vi "add to buffer.vi"(10 "read data":string, 11 "buffer in":cluster{"data":u8[], "packets contained":i32}[](array[cluster])) -> (3 "buffer out":cluster{"data":u8[], "packets contained":i32}[](array[cluster]))   [LabVIEW 2020, in "SubVIs.lvlib" / "RTU Data Unit.lvclass"]
uses:
  <vilib>/Modbus/subvis/Transmission Data Unit (ADU)/RTU Data Unit/RTU Data Unit.lvclass
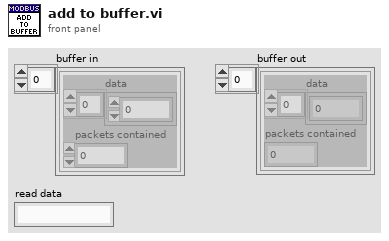
[diagram p1: front panel]
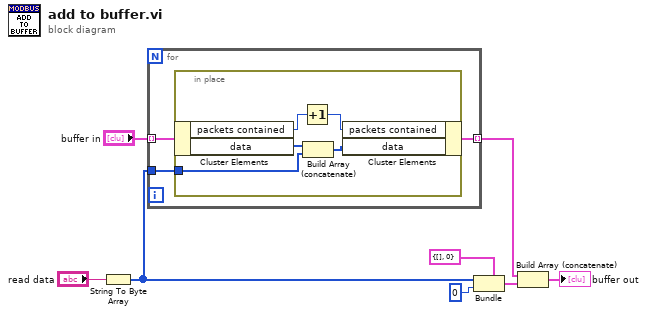
[diagram p0: block diagram]
diagram:
  n1 = String To Byte Array(string="read data") -> (unsigned byte array=w3:u8[])
  n2 = for {
    tunnel: "buffer in" -> [w11] mode=indexing
    tunnel: [w10] -> w4 mode=indexing
    tunnel: w3 -> [w9]
    n3 = in-place {
      in-place-border: w9 -> [w14]
      n4 = in-place-cluster #1(w11) -> ("packets contained"=w13:i32, "data"=w16:u8[])
      n5 = Increment(x=w13) -> (x+1=w12:i32)
      n6 = Build Array (concatenate)(w16, w14) -> (w15:u8[])
      n7 = in-place-cluster #1("packets contained"=w12, "data"=w15) -> (w10:cluster{"data":u8[], "packets contained":i32})
    }
  }
  n8 = Bundle(cluster=cluster{"data":u8[], "packets contained":i32} {"data"=[], "packets contained"=0}, "data"=w3, "packets contained"=0) -> (w6:cluster{"data":u8[], "packets contained":i32})
  n9 = Build Array (concatenate)(w4, w6) -> (→"buffer out":cluster{"data":u8[], "packets contained":i32}[])
